vi "Configure.vi"(8 "error in (no error)":errorcluster, 11 "Galvo in":refnum<class "InVivo_ImagingModeSPIM.lvclass">) -> (0 "error out":errorcluster, 2 "cancelled?":bool=TRUE, 3 "Galvo out":refnum<class "InVivo_ImagingModeSPIM.lvclass">)   [LabVIEW 2012, in "InVivo_ImagingModeSPIM.lvclass"]
doc: "The configure method configures the details for the RabbitMQ connection. \n\nIn the derived class, make a call to the parent for setting these parameters."
uses:
  InVivo_ImagingModeSPIM.lvclass
  <vilib>/Utility/miscctls.llb/LVPointTypeDef.ctl
  InVivo_ImagingModeSPIM.lvclass/InVivo_ImagingModeSPIM.ctl
  <vilib>/Distrio/Murmex/Murmex/Murmex.lvclass
panel:
  in  "No. channels":u8
  in  "Sampling rate":dbl=10000.0 format="%#_6e"
  in  "Samples/channel":i32=1000
  in  "button::cancel":bool
  in  "button::ok":bool
  in  "button::configure murmex":bool
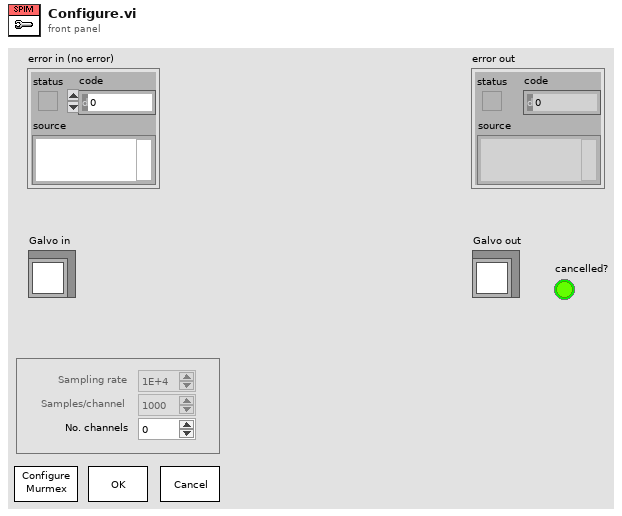
[diagram p1: front panel]
types:
  T1 = typedef "LVPointTypeDef.ctl" = cluster{"Horizontal":i16, "Vertical":i16}
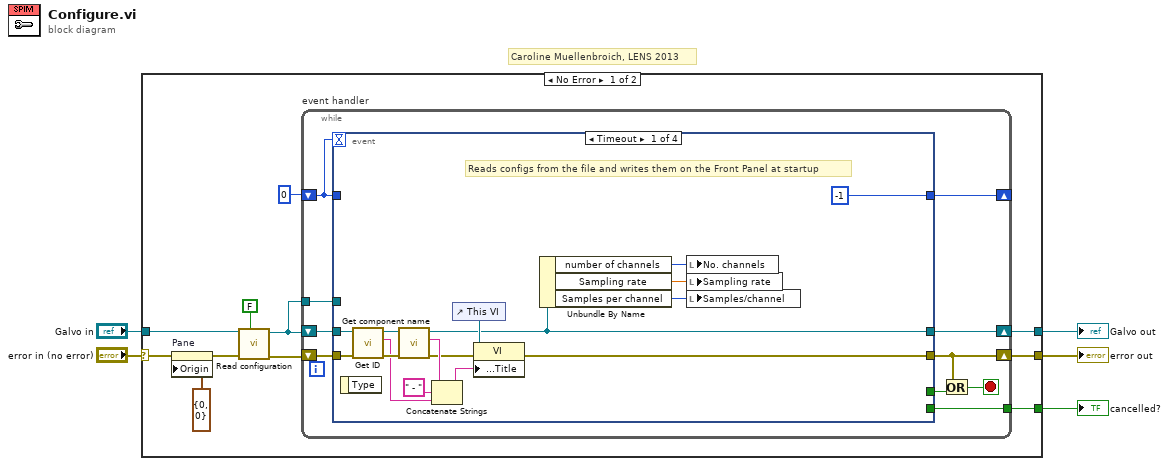
[diagram p0: block diagram]
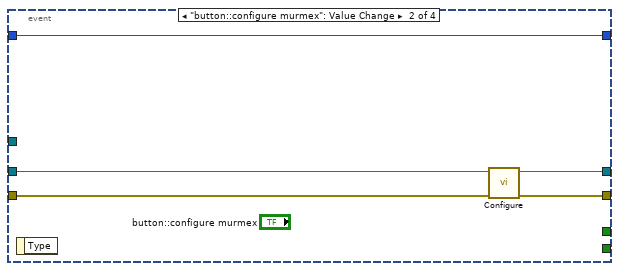
[diagram p2: hidden frame]
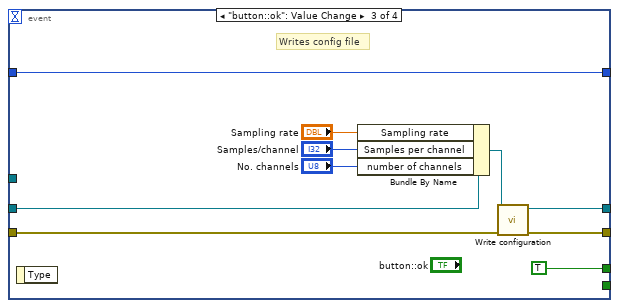
[diagram p3: hidden frame]
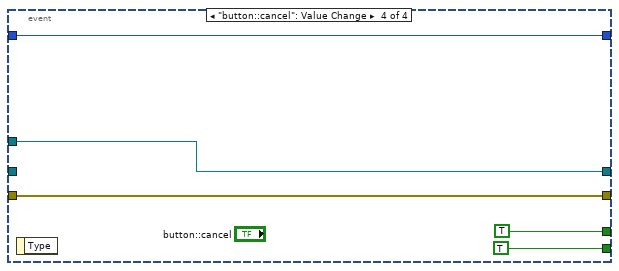
[diagram p4: hidden frame]
diagram:
  # "Caroline Muellenbroich, LENS 2013"
  n1 = case shown="No Error" "error in (no error)" {
    selector: "error in (no error)" -> [w10 w64]
    tunnel: [w15 _] -> w5
    tunnel: [w14 w63] -> w4
    tunnel: [w13 w64] -> w3
    tunnel: "Galvo in" -> [w11 w63]
    frame No Error {
      n2 = property on="Pane" class="Pane"(error in=w10, "Origin"=T1 {"Horizontal"=0, "Vertical"=0}) -> (error out=w8:errorcluster)  [unwired: 1 in, 1 out]
      n3 = call-dynamic "Read configuration.vi"("force loading?"=FALSE, "error in (no error)"=w8, "Galvo in"=w11) -> ("error out"=w7:errorcluster, "Galvo out"=w6:refnum<class "InVivo_ImagingModeSPIM.lvclass">)  [unwired: 7 in]
      n4 = while "event handler" {
        shift-right: [w26] -> _
        shift-left: 0 -> [w17]
        shift-right: [w23] -> w14
        shift-left: w6 -> [w24]
        shift-right: [w22] -> w13
        shift-left: w7 -> [w25]
        tunnel: [w19] -> w15
        tunnel: w6 -> [w18]
        stop <- w20 stop-if-true
        n5 = event shown="[0] Timeout" {
          selector: _ -> [_ _ _ _]
          dyn-events: _ -> [_ _ _ _]
          timeout: w17 -> [_ _ _ _]
          tunnel: w17 -> [_ w43 w51 w59]
          tunnel: [-1 w43 w51 w59] -> w26
          tunnel: w25 -> [w37 w46 w53 w62]
          tunnel: w24 -> [w41 w47 w55 _]
          tunnel: [w29 w45 w57 w58] -> w23
          tunnel: [w28 w44 w56 w62] -> w22
          tunnel: [_ _ TRUE ("force loading?") TRUE ("force loading?")] -> w21
          tunnel: [_ _ _ TRUE ("force loading?")] -> w19
          tunnel: w18 -> [_ _ _ w58]
          event Timeout {
            # "Reads configs from the file and writes them on the Front Panel at startup"
            n6 = event-data() -> ()  [unwired: 1 in, 1 out]
            n7 = call <vilib>:"Get ID.vi"("error in (no error)"=w37, "Murmex in"=w41) -> ("error out"=w36:errorcluster, "component id"=w32:string, "Murmex out"=w35:refnum<class "InVivo_ImagingModeSPIM.lvclass">)  [unwired: 7 in]
            n8 = call <vilib>:"Get component name.vi"("error in (no error)"=w36, "Murmex in"=w35) -> ("error out"=w30:errorcluster, "component name"=w31:string, "Murmex out"=w29:refnum<class "InVivo_ImagingModeSPIM.lvclass">)  [unwired: 7 in]
            n9 = Concatenate Strings(w31, " - " ("string"), w32) -> (w33:string)
            n10 = control-ref of="This VI"() -> (w38:refnum<vi>)
            n11 = property class="VI"(reference=w38, error in=w30, "Front Panel.Title"=w33) -> (error out=w28:errorcluster)  [unwired: 1 out]
            n12 = Unbundle By Name(w29) -> ("number of channels"=w27:u8, "Sampling rate"=w40:dbl, "Samples per channel"=w39:i32)
            n13 = local write "No. channels"(w27) -> ()
            n14 = local write "Sampling rate"(w40) -> ()
            n15 = local write "Samples/channel"(w39) -> ()
          }
          event "button::configure murmex": Value Change {
            n16 = event-data() -> ()  [unwired: 1 in, 1 out]
            n17 = call-parent "Configure.vi"("error in (no error)"=w46, "Murmex in"=w47) -> ("error out"=w44:errorcluster, "Murmex out"=w45:refnum<class "InVivo_ImagingModeSPIM.lvclass">)  [unwired: 7 in, 1 out]
          }
          event "button::ok": Value Change {
            # "Writes config file"
            n18 = event-data() -> ()  [unwired: 1 in, 1 out]
            n19 = Bundle By Name(cluster=w55, "Sampling rate"="Sampling rate", "Samples per channel"="Samples/channel", "number of channels"="No. channels") -> (w54:refnum<class "InVivo_ImagingModeSPIM.lvclass">)
            n20 = call-dynamic "Write configuration.vi"("error in (no error)"=w53, "Galvo in"=w54) -> ("error out"=w56:errorcluster, "Galvo out"=w57:refnum<class "InVivo_ImagingModeSPIM.lvclass">)  [unwired: 8 in]
          }
          event "button::cancel": Value Change {
            n21 = event-data() -> ()  [unwired: 1 in, 1 out]
          }
        }
        n22 = Or(x=w22, y=w21) -> (x .or. y?=w20:bool)
      }
    }
    frame Error {
    }
  }
  "error out" <- w3
  "Galvo out" <- w4
  "cancelled?" <- w5
